vi "Returning Values By Reference Array Of Complex Struct Corrected.vi"() -> ()   [LabVIEW 2009, in "LabVIEWWrapper_PassingDataSampleDLL.lvlib"]
doc: "void ReturningValuesByReference_ArrayOfComplexStruct (struct complexStructPolygon **triangles, int length);"
uses:
  LabVIEWWrapper_PassingDataSampleDLL.lvlib
  CustomControlsForStructs/ComplexStruct Polygon.ctl
  PassingDataSampleDLL.dll
panel:
  out "Triangle":T1[](array[typedef])
  out "Pointer to Array of Triangles":i64
  out "error out":errorcluster
  in  "error in (no error)":errorcluster
  in  "length":i32
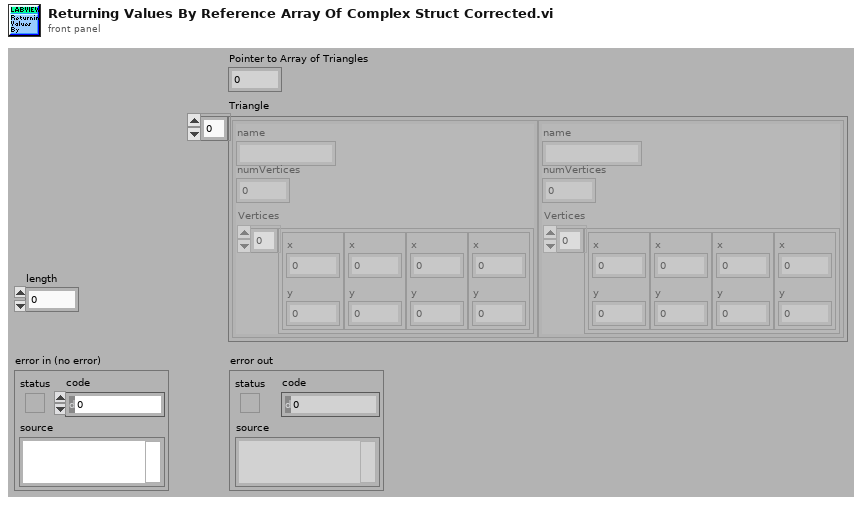
[diagram p1: front panel]
types:
  T1 = typedef "LabVIEWWrapper_PassingDataSampleDLL.lvlib/ComplexStruct Polygon.ctl" = cluster{"name":string, "numVertices":i32, "Vertices":cluster{"x":i32, "y":i32}[]}
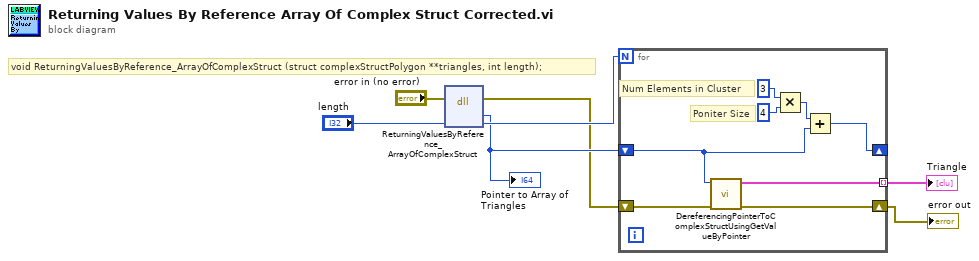
[diagram p0: block diagram]
diagram:
  # "void ReturningValuesByReference_ArrayOfComplexStruct (struct complexStructPolygon **triangles, int length);"
  n1 = dll-call lib="C:/My Dropbox/Systems Engineering Application/SDK/C Integration/LabVIEWWrapper/PassingDataSampleDLL.*" fn="ReturningValuesByReference_ArrayOfComplexStruct"(error in="error in (no error)", "length"="length") -> (error out=w2:errorcluster, "triangles"=w4:i64, "length"=w5:i32)  [unwired: 4 in, 1 out]
  "Pointer to Array of Triangles" <- w4
  n2 = for {
    N: w5 -> [_]
    shift-right: [w15] -> _
    shift-left: w4 -> [w14]
    tunnel: [w13] -> w3 mode=indexing
    shift-right: [w11] -> w1
    shift-left: w2 -> [w12]
    # "Poniter Size"
    # "Num Elements in Cluster"
    n3 = call "DereferencingPointerToComplexStructUsingGetValueByPointer.vi"("error in (no error)"=w12, "Pointer"=w14) -> ("error out"=w11:errorcluster, "ComplexStruct Polygon"=w13:T1)  [unwired: 8 in]
    n4 = Multiply(x=3, y=4) -> (x*y=w8:i32)
    n5 = Add(x=w8, y=w14) -> (x+y=w15:i64)
  }
  "error out" <- w1
  "Triangle" <- w3
